vi "MGCC_Resync_main.vi"() -> ()   [LabVIEW 2016]
uses:
  <vilib>/Utility/error.llb/Error Cluster From Error Code.vi
  Communication/Global communication.vi
  Model Management/Global_MdlMgmt.vi
  MGCC_Resync_global.vi
  Communication/Global communication output.vi
  Finite State Machine/Sub-VIs/MGCC_FntStaMach_gobal.vi
  <vilib>/ErrorRing/Error Ring.xnode
panel:
  out "b_MGCC_FntStaMach_All_Loop_Stop":bool
  out "Resync Iterations":i16
  # "Copyright <2020> <The University of Tennessee at Knoxville and the University of Tennessee Research Foundation>\n\nRedistribution and use in source and binary forms, with or without modification, are permitted provided that the following conditions are met:\n\n1. Redistributions of source code must retain the above copyright notice, this list of conditions and the following disclaimer.\n\n2. Redistributions in binary form must reproduce the above copyright notice, this list of conditions and the following disclaimer in the documentation and/or other materials provided with the distribution.\n\n3. Neither the name of the copyright holder nor the names of its contributors may be used to endorse or promote products derived from this software without specific prior written permission.\n\nTHIS SOFTWARE IS PROVIDED BY THE COPYRIGHT HOLDERS AND CONTRIBUTORS \"AS IS\" AND ANY EXPRESS OR IMPLIED WARRANTIES, INCLUDING, BUT NOT LIMITED TO, THE IMPLIED WARRANTIES OF MERCHANTABILITY AND FITNESS FOR A PARTICULAR PURPOSE ARE DISCLAIMED. IN NO EVENT SHALL THE COPYRIGHT HOLDER OR CONTRIBUTORS BE LIABLE FOR ANY DIRECT, INDIRECT, INCIDENTAL, SPECIAL, EXEMPLARY, OR CONSEQUENTIAL DAMAGES (INCLUDING, BUT NOT LIMITED TO, PROCUREMENT OF SUBSTITUTE GOODS OR SERVICES; LOSS OF USE, DATA, OR PROFITS; OR BUSINESS INTERRUPTION) HOWEVER CAUSED AND ON ANY THEORY OF LIABILITY, WHETHER IN CONTRACT, STRICT LIABILITY, OR TORT (INCLUDING NEGLIGENCE OR OTHERWISE) ARISING IN ANY WAY OUT OF THE USE OF THIS SOFTWARE, EVEN IF ADVISED OF THE POSSIBILITY OF SUCH DAMAGE."
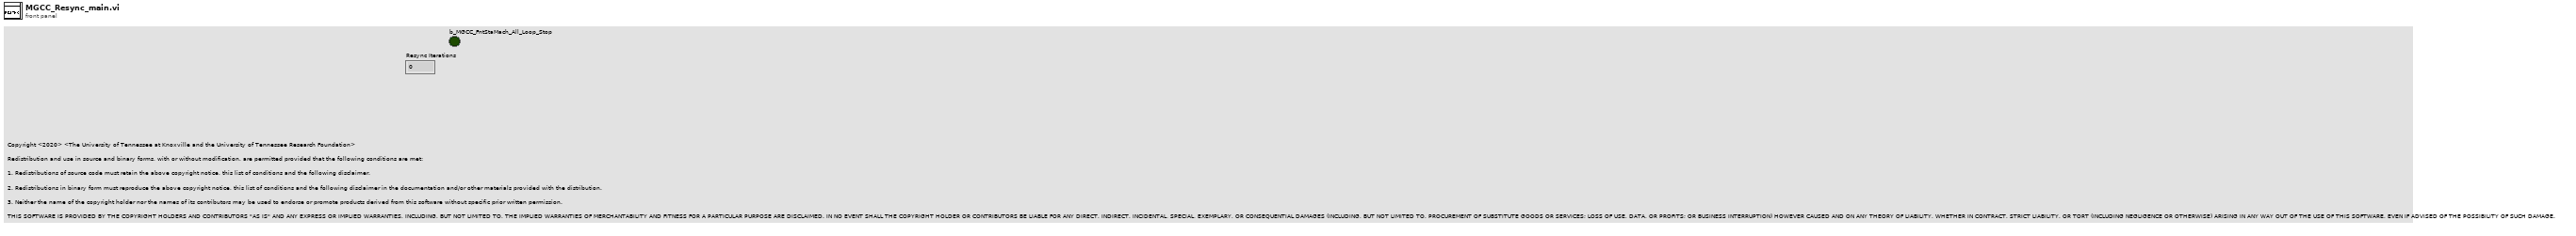
[diagram p1: front panel]
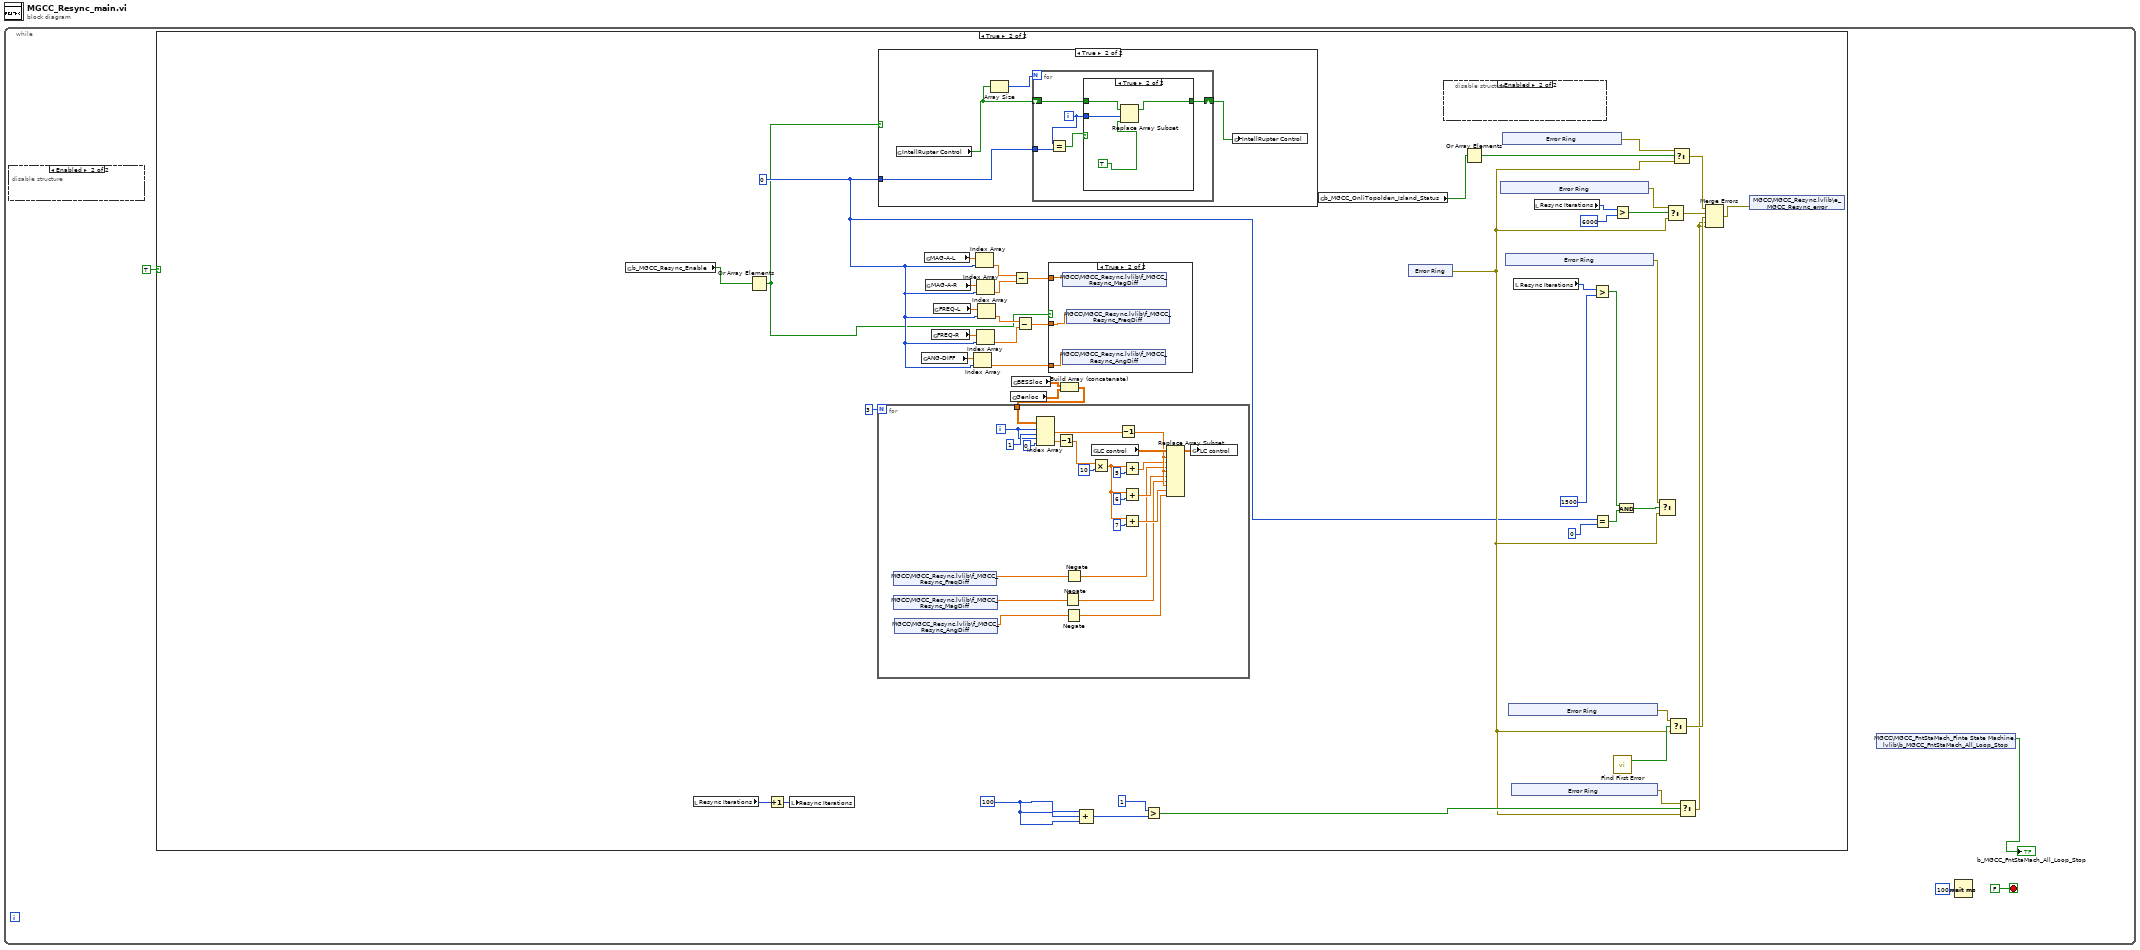
[diagram p0: block diagram]
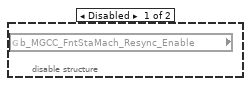
[diagram p2: hidden frame]
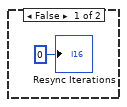
[diagram p3: hidden frame]
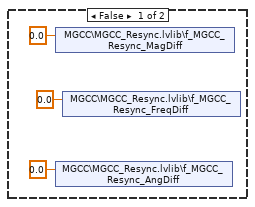
[diagram p6: hidden frame]
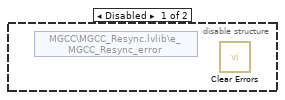
[diagram p7: hidden frame]
diagram:
  n1 = while {
    stop <- FALSE stop-if-true
    n2 = disable-structure shown="Enabled" {
      frame Disabled {
        n3 = global read "MGCC_FntStaMach_gobal.vi" "b_MGCC_FntStaMach_Resync_Enable"() -> ()  [unwired: 1 out]
      }
      frame Enabled {
      }
    }
    n4 = case shown="True" TRUE {
      frame False {
        "Resync Iterations" <- i16 0 ("Resync Iterations")
      }
      frame True {
        w11 = 0
        w33 = 100 ("y")
        n5 = global read "MGCC_Resync_global.vi" "b_MGCC_Resync_Enable"() -> (w12:bool[])
        n6 = local read "Resync Iterations"() -> (w53:i16)
        n7 = Or Array Elements(Boolean array=w12) -> (logical OR=w6:bool)
        n8 = Increment(x=w53) -> (x+1=w52:i16)
        n9 = local write "Resync Iterations"(w52) -> ()
        n10 = case shown="True" w6 {
          tunnel: w11 -> [_ w57]
          frame False {
          }
          frame True {
            n11 = global read "Global communication output.vi" "IntellRupter Control"() -> (w56:bool[])
            n12 = Array Size(array=w56) -> (size(s)=w55:i32)
            n13 = for {
              N: w55 -> [_]
              shift-right: [w61] -> w54
              shift-left: w56 -> [w62]
              tunnel: w57 -> [w58]
              i -> [w60]
              n14 = Equal?(x=w60, y=w58) -> (x = y?=w59:bool)
              n15 = case shown="True" w59 {
                tunnel: w62 -> [w63 w67]
                tunnel: w60 -> [_ w66]
                tunnel: [w63 w65] -> w61
                frame False {
                }
                frame True {
                  n16 = Replace Array Subset(array=w67, new element=TRUE ("new element/subarray"), index=w66) -> (w65:bool[])
                }
              }
            }
            n17 = global write "Global communication output.vi" "IntellRupter Control"(w54) -> ()
          }
        }
        n18 = global read "Global communication.vi" "ANG-DIFF"() -> (w21:dbl[])
        n19 = global read "Global communication.vi" "MAG-A-L"() -> (w25:dbl[])
        n20 = global read "Global communication.vi" "MAG-A-R"() -> (w24:dbl[])
        n21 = global read "Global communication.vi" "FREQ-R"() -> (w22:dbl[])
        n22 = global read "Global communication.vi" "FREQ-L"() -> (w23:dbl[])
        n23 = Index Array(array=w21, index=w11) -> (element=w26:dbl)
        n24 = Index Array(array=w25, index=w11) -> (element=w20:dbl)
        n25 = Index Array(array=w24, index=w11) -> (element=w19:dbl)
        n26 = Index Array(array=w22, index=w11) -> (element=w17:dbl)
        n27 = Index Array(array=w23, index=w11) -> (element=w18:dbl)
        n28 = global read "Global_MdlMgmt.vi" "Genloc"() -> (w14:dbl[][])
        n29 = global read "Global_MdlMgmt.vi" "BESSloc"() -> (w15:dbl[][])
        n30 = Subtract(x=w20, y=w19) -> (x-y=w16:dbl)
        n31 = Subtract(x=w18, y=w17) -> (x-y=w27:dbl)
        n32 = case shown="True" w6 {
          tunnel: w27 -> [_ w73]
          tunnel: w26 -> [_ w72]
          tunnel: w16 -> [_ w71]
          frame False {
            n33 = shared-variable "MGCC\\MGCC_Resync.lvlib\\f_MGCC_Resync_MagDiff"(0.0 ("f_MGCC_Resync_MagDiff")) -> ()  [unwired: 1 in, 1 out]
            n34 = shared-variable "MGCC\\MGCC_Resync.lvlib\\f_MGCC_Resync_AngDiff"(0.0 ("f_MGCC_Resync_AngDiff")) -> ()  [unwired: 1 in, 1 out]
            n35 = shared-variable "MGCC\\MGCC_Resync.lvlib\\f_MGCC_Resync_FreqDiff"(0.0 ("f_MGCC_Resync_FreqDiff")) -> ()  [unwired: 1 in, 1 out]
          }
          frame True {
            n36 = shared-variable "MGCC\\MGCC_Resync.lvlib\\f_MGCC_Resync_MagDiff"(w71) -> ()  [unwired: 1 in, 1 out]
            n37 = shared-variable "MGCC\\MGCC_Resync.lvlib\\f_MGCC_Resync_AngDiff"(w72) -> ()  [unwired: 1 in, 1 out]
            n38 = shared-variable "MGCC\\MGCC_Resync.lvlib\\f_MGCC_Resync_FreqDiff"(w73) -> ()  [unwired: 1 in, 1 out]
          }
        }
        n39 = Build Array (concatenate)(w15, w14) -> (w13:dbl[][])
        n40 = for {
          N: 3 -> [_]
          tunnel: w13 -> [w92]
          i -> [w77]
          n41 = shared-variable "MGCC\\MGCC_Resync.lvlib\\f_MGCC_Resync_FreqDiff"() -> (w96:dbl)  [unwired: 1 in, 1 out]
          n42 = shared-variable "MGCC\\MGCC_Resync.lvlib\\f_MGCC_Resync_MagDiff"() -> (w97:dbl)  [unwired: 1 in, 1 out]
          n43 = shared-variable "MGCC\\MGCC_Resync.lvlib\\f_MGCC_Resync_AngDiff"() -> (w95:dbl)  [unwired: 1 in, 1 out]
          n44 = Index Array(array=w92, index (row) #1=w77, index (col) #1=1 ("disabled index (col)"), index (row) #2=w77, index (col) #2=0 ("disabled index (col)")) -> (element #1=w88:dbl, element #2=w87:dbl)
          n45 = Decrement(x=w87) -> (x-1=w86:dbl)
          n46 = Negate(x=w97) -> (-x=w75:dbl)
          n47 = Negate(x=w95) -> (-x=w74:dbl)
          n48 = Negate(x=w96) -> (-x=w76:dbl)
          n49 = global read "Global communication.vi" "LC control"() -> (w94:dbl[][])
          n50 = Multiply(x=w86, y=10 ("disabled index (col)")) -> (x*y=w80:dbl)
          n51 = Decrement(x=w88) -> (x-1=w89:dbl)
          n52 = Add(x=w80, y=5 ("disabled index (col)")) -> (x+y=w84:dbl)
          n53 = Add(x=w80, y=6 ("disabled index (col)")) -> (x+y=w83:dbl)
          n54 = Add(x=w80, y=7 ("disabled index (col)")) -> (x+y=w82:dbl)
          n55 = Replace Array Subset(array=w94, new element #1=w76, index (row) #1=w89, index (col) #1=w84, new element #2=w75, index (row) #2=w89, index (col) #2=w83, new element #3=w74, index (row) #3=w89, index (col) #3=w82) -> (w93:dbl[][])
          n56 = global write "Global communication.vi" "LC control"(w93) -> ()
        }
        n57 = Compound Arithmetic op=unknown(w33, w33, w33) -> (w32:i32)
        n58 = Greater?(x=1 ("y"), y=w32) -> (0:w30:bool)
        n59 = global read "MGCC_FntStaMach_gobal.vi" "b_MGCC_OnliTopolden_Island_Status"() -> (w10:bool[])
        n60 = xnode "Error Ring"() -> ("error out"=w28:errorcluster)
        n61 = disable-structure shown="Enabled" {
          frame Disabled {
            n62 = shared-variable "MGCC\\MGCC_Resync.lvlib\\e_MGCC_Resync_error"() -> ()  [unwired: 1 in, 2 out]
            n63 = call <vilib>:"Clear Errors.vi"() -> ()  [unwired: 6 in, 2 out]
          }
          frame Enabled {
          }
        }
        n64 = Or Array Elements(Boolean array=w10) -> (logical OR=w9:bool)
        n65 = xnode "Error Ring"() -> ("error out"=w48:errorcluster)
        n66 = xnode "Error Ring"() -> ("error out"=w47:errorcluster)
        n67 = xnode "Error Ring"() -> ("error out"=w34:errorcluster)
        n68 = xnode "Error Ring"() -> ("error out"=w45:errorcluster)
        n69 = xnode "Error Ring"() -> ("error out"=w29:errorcluster)
        n70 = local read "Resync Iterations"() -> (w39:i16)
        n71 = local read "Resync Iterations"() -> (w51:i16)
        n72 = Greater?(x=w39, y=i16 1500) -> (0:w37:bool)
        n73 = Equal?(x=w11, y=i16 0) -> (x = y?=w36:bool)
        n74 = Greater?(x=w51, y=i16 6000) -> (0:w49:bool)
        n75 = call <vilib>:"Find First Error.vi"() -> ("error?"=w46:bool)  [unwired: 4 in, 1 out]
        n76 = And(x=w37, y=w36) -> (x .and. y?=w35:bool)
        n77 = Select(t=w34, s=w35, f=w28) -> ()  [unwired: 1 out]
        n78 = Select(t=w48, s=w49, f=w28) -> (s? t:f=w43:errorcluster)
        n79 = Select(t=w45, s=w46, f=w28) -> (s? t:f=w42:errorcluster)
        n80 = Select(t=w47, s=w9, f=w28) -> (s? t:f=w44:errorcluster)
        n81 = Select(t=w29, s=w30, f=w28) -> (s? t:f=w7:errorcluster)
        n82 = Merge Errors(w44, w43, w42, w7, w7) -> (w41:errorcluster)
        n83 = shared-variable "MGCC\\MGCC_Resync.lvlib\\e_MGCC_Resync_error"(error in=w41) -> ()  [unwired: 2 out]
      }
    }
    n84 = shared-variable "MGCC\\MGCC_FntStaMach_Finte State Machine.lvlib\\b_MGCC_FntStaMach_All_Loop_Stop"() -> (→"b_MGCC_FntStaMach_All_Loop_Stop":bool)  [unwired: 1 in, 1 out]
    n85 = Wait (ms)(milliseconds to wait=u32 100) -> ()  [unwired: 1 out]
  }
